vi "I2C Bus Monitor Test.vi"() -> ()   [LabVIEW 2025]
uses:
  b35e104c-1675-4f6f-8f1c-29597b7e93d1.vi
  I2C Bus Monitor UI/I2C Bus Monitor UI.lvlib
  I2C Bus Monitor/I2C Bus Monitor.lvclass
panel:
  out "Count":i32
  in  "Select 2":bool
  in  "SERIAL INPUT (SI)":u32(ring)
  in  "Select":bool
  in  "RESOURCE NAME":u32(ring)
  in  "I2C Scrpit Path":path
  in  "Serial Channel":string(combo)
  in  "Send I2C Script":bool
  out "I2C Script Error":errorcluster
  out "I2C Transaction Error":errorcluster
  in  "I2C Command":T1 {"Data" format="%02x"; "Register Address" format="%04x"; "Slave Address" format="%02x"}
  out "Read Data":u8 format="%02x"
  in  "Send I2C Transaction":bool
  out "User Timestamp Fifo Overflow":bool
  out "i":i32
  out "I2C Messages":string[][](table)
  out "Total Messages":i32
  out "FIFO Pressure":u32
  in  "stop":bool
  out "Bitfile Path":path
  out "SI Count":i32
  out "Module Name":string
  out "error out":errorcluster
  # "takes few seconds to populate"
  # "1"
  # "2"
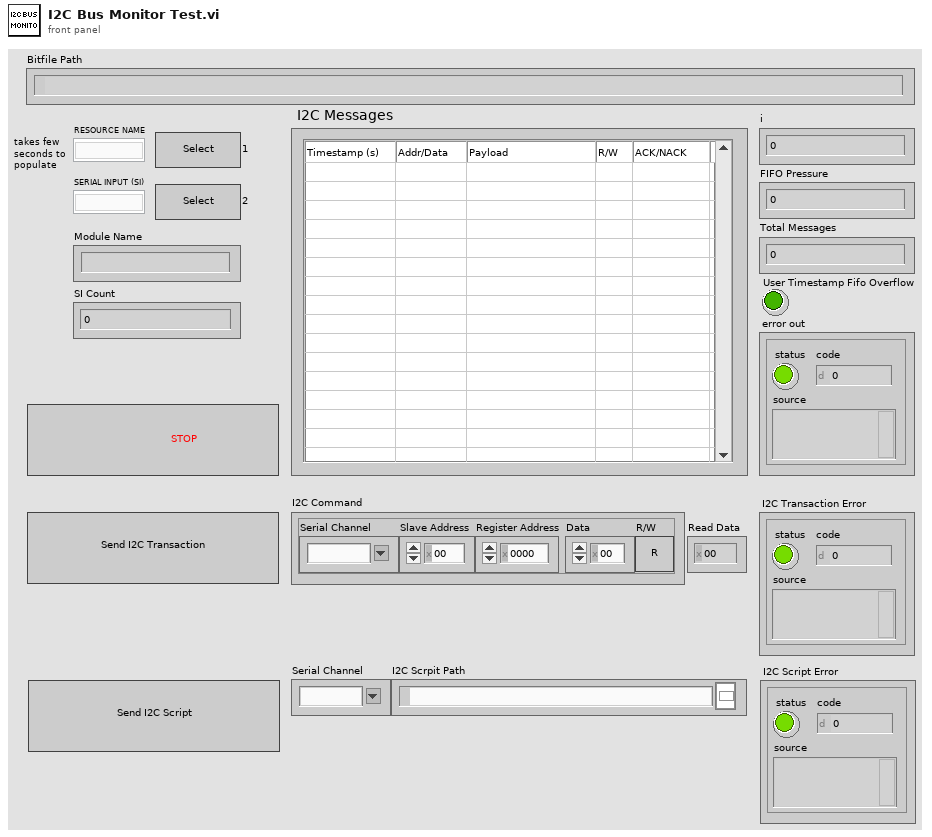
[diagram p1: front panel]
types:
  T1 = cluster{"Serial Channel":string, "Slave Address":u8, "Register Address":u16, "Data":u8, "R/W":bool}
  T2 = typedef "NI CSI-2 API FPGA v2.lvlib/Timestamp ID.ctl" = enum8{"SI0 LLP", "SI1 LLP", "SI2 LLP", "SI3 LLP", "SI4 LLP", "SI5 LLP", "SI6 LLP", "SI7 LLP", "SO0 LLP", "SO1 LLP", "SO2 LLP", "SO3 LLP", "SO4 LLP", "SO5 LLP", "SO6 LLP", "SO7 LLP", "Ser0 GPIO Bank", "Ser1 GPIO Bank", "Ser2 GPIO Bank", "Ser3 GPIO Bank", "Ser4 GPIO Bank", "Ser5 GPIO Bank", "Ser6 GPIO Bank", "Ser7 GPIO Bank", "Des0 GPIO Bank", "Des1 GPIO Bank", "Des2 GPIO Bank", "Des3 GPIO Bank", "Des4 GPIO Bank", "Des5 GPIO Bank", "Des6 GPIO Bank", "Des7 GPIO Bank", "User0", "User1", "User2", "User3", "User4", "User5", "User6", "User7", "User8", "User9", "User10", "User11", "User12", "User13", "User14", "User15", "User16", "User17", "User18", "User19", "User20", "User21", "User22", "User23", "User24", "User25", "User26", "User27", "User28", "User29", "User30", "User31"}
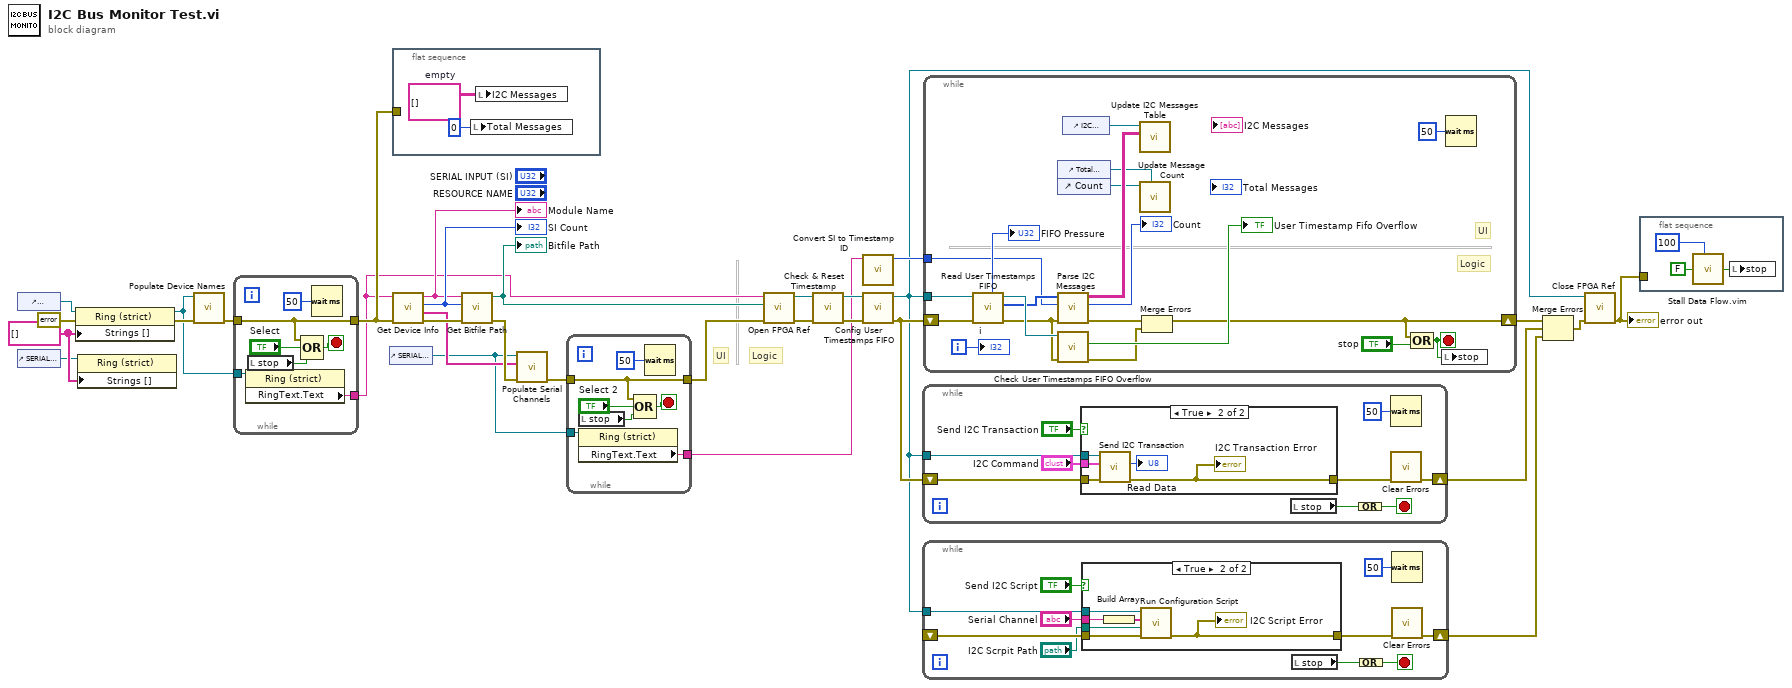
[diagram p0: block diagram]
diagram:
  w2 = string[] [] ("Strings []")
  # "Logic"
  # "UI"
  n1 = control-ref of="RESOURCE NAME"() -> (w4:refnum<vi>)
  n2 = control-ref of="SERIAL INPUT (SI)"() -> (w1:refnum<vi>)
  n3 = property class="Ring (strict)"(reference=w4, error in=errorcluster {"status"=FALSE, "code"=0, "source"=""} ("error constant"), "Strings []"=w2) -> (reference out=w3:refnum<vi>, error out=w5:errorcluster)
  n4 = property class="Ring (strict)"(reference=w1, "Strings []"=w2) -> ()  [unwired: 1 in, 2 out]
  n5 = call "Populate Device Names.vi"("error in (no error)"=w5, "RESOURCE NAME Ref"=w3) -> ("error out"=w14:errorcluster)  [unwired: 8 in, 1 out]
  n6 = while {
    tunnel: [w35] -> w15
    tunnel: w14 -> [w35]
    tunnel: w3 -> [w34]
    tunnel: [w33] -> w6
    stop <- w36 stop-if-true
    n7 = property class="Ring (strict)"(reference=w34) -> ("RingText.Text"=w33:string)  [unwired: 1 in, 2 out]
    n8 = local read "stop"() -> (w32:bool)
    n9 = Compound Arithmetic op=OR(w35, "Select", w32) -> (w36:bool)
    n10 = Wait (ms)(milliseconds to wait=u32 50) -> ()  [unwired: 1 out]
  }
  n11 = control-ref of="SERIAL INPUT (SI)"() -> (w9:refnum<vi>)
  n12 = flat-sequence {
    tunnel: w15 -> [_]
    frame #0 {
      w40 = string[][] []  # empty
      n13 = local write "Total Messages"(0 ("Total Records out")) -> ()
      n14 = local write "I2C Messages"(w40) -> ()
    }
  }
  n15 = call "Get Device Info.vi"("error in (no error)"=w15, "RIO Device"=w6) -> ("error out"=w31:errorcluster, "SI Channels"=w12:string[], "SI Count"=w30:i32, "Module Name"=w13:string)  [unwired: 6 in]
  "Module Name" <- w13
  "SI Count" <- w30
  n16 = call "Get Bitfile Path.vi"("error in (no error)"=w31, "SI Count"=w30, "Module Name"=w13) -> ("error out"=w26:errorcluster, "Bitfile Path"=w29:path)  [unwired: 7 in]
  "Bitfile Path" <- w29
  n17 = call "Populate Serial Channels.vi"("error in (no error)"=w26, "Strings []"=w12, "SERIAL INPUT (SI) Ref in"=w9) -> ("error out"=w11:errorcluster)  [unwired: 7 in, 1 out]
  n18 = while {
    tunnel: [w45] -> w10
    tunnel: w11 -> [w45]
    tunnel: w9 -> [w44]
    tunnel: [w43] -> w7
    stop <- w46 stop-if-true
    n19 = local read "stop"() -> (w41:bool)
    n20 = property class="Ring (strict)"(reference=w44) -> ("RingText.Text"=w43:string)  [unwired: 1 in, 2 out]
    n21 = Compound Arithmetic op=OR(w45, "Select 2", w41) -> (w46:bool)
    n22 = Wait (ms)(milliseconds to wait=u32 50) -> ()  [unwired: 1 out]
  }
  n23 = call "Open FPGA Ref.vi"("error in (no error)"=w10, "Bitfile Path"=w29, "Device address"=w6) -> ("error out"=w28:errorcluster, "FPGA Ref out"=w20:refnum<k20>)  [unwired: 7 in]
  n24 = call "Check & Reset Timestamp.vi"("error in (no error)"=w28, "FPGA Ref in"=w20) -> ("error out"=w21:errorcluster, "FPGA Ref out"=w19:refnum<k20>)  [unwired: 8 in]
  n25 = call "Convert SI to Timestamp ID.vi"("SI Channel"=w7) -> ("Timestamp ID"=w25:T2)  [unwired: 10 in]
  n26 = call "Config User Timestamps FIFO.vi"("error in (no error)"=w21, "FPGA Ref in"=w19) -> ("error out"=w24:errorcluster, "FPGA Ref out"=w18:refnum<k20>)  [unwired: 8 in]
  n27 = while {
    tunnel: w18 -> [w50]
    shift-right: [w48] -> w22
    shift-left: w24 -> [w54]
    stop <- w56 stop-if-true
    n28 = case shown="True" "Send I2C Transaction" {
      tunnel: w54 -> [w57 w62]
      tunnel: [w57 w58] -> w49
      tunnel: "I2C Command" -> [_ w61]
      tunnel: w50 -> [_ w59]
      frame False {
      }
      frame True {
        n29 = call "Send I2C Transaction.vi"("Error In"=w62, "I2C Command"=w61, "FPGA Ref in"=w59) -> ("Error Out"=w58:errorcluster, "Read Data"=→"Read Data":u8)  [unwired: 6 in, 1 out]
        "I2C Transaction Error" <- w58
      }
    }
    n30 = local read "stop"() -> (w55:bool)
    n31 = Compound Arithmetic op=OR(w55) -> (w56:bool)
    n32 = Wait (ms)(milliseconds to wait=u32 50) -> ()  [unwired: 1 out]
    n33 = call <vilib>:"Clear Errors.vi"("error in (no error)"=w49) -> ("error out"=w48:errorcluster)  [unwired: 5 in, 1 out]
  }
  n34 = while {
    shift-right: [w66] -> w17
    shift-left: _ -> [w70]
    tunnel: w18 -> [w65]
    stop <- w72 stop-if-true
    n35 = case shown="True" "Send I2C Script" {
      tunnel: w70 -> [w73 w79]
      tunnel: [w73 w77] -> w67
      tunnel: w65 -> [_ w78]
      tunnel: "I2C Scrpit Path" -> [_ w76]
      tunnel: "Serial Channel" -> [_ w75]
      frame False {
      }
      frame True {
        n36 = Build Array(w75) -> (w74:string[])
        n37 = call "Run Configuration Script.vi"("error in (no error)"=w79, "configuration script"=w76, "serial channels"=w74, "fpga interface in"=w78) -> ("error out"=w77:errorcluster)  [unwired: 6 in, 1 out]
        "I2C Script Error" <- w77
      }
    }
    n38 = local read "stop"() -> (w71:bool)
    n39 = Compound Arithmetic op=OR(w71) -> (w72:bool)
    n40 = Wait (ms)(milliseconds to wait=u32 50) -> ()  [unwired: 1 out]
    n41 = call <vilib>:"Clear Errors.vi"("error in (no error)"=w67) -> ("error out"=w66:errorcluster)  [unwired: 5 in, 1 out]
  }
  n42 = while {
    shift-right: [w86] -> w27
    shift-left: w24 -> [w97]
    tunnel: w25 -> [w83]
    tunnel: w18 -> [w98]
    i -> [w96]
    stop <- w84 stop-if-true
    # "Logic"
    # "UI"
    n43 = call "Read User Timestamps FIFO.vi"("error in (no error)"=w97, "FPGA Ref in"=w98) -> ("error out"=w89:errorcluster, "Data"=w90:u64[], "FPGA Ref out"=w93:refnum<k20>, "Elements Remaining"=→"FIFO Pressure":u32)  [unwired: 6 in]
    n44 = control-ref of="Total Messages"() -> (w82:refnum<vi>)
    n45 = control-ref of="Count"() -> (w80:refnum<vi>)
    n46 = call "Parse I2C Messages.vi"("error in (no error)"=w89, "Timestamp ID"=w83, "User Timestamps"=w90) -> ("error out"=w88:errorcluster, "Count"=→"Count":i32, "I2C Messages"=w85:string[][])  [unwired: 6 in]
    n47 = call "Check User Timestamps FIFO Overflow.vi"("error in (no error)"=w89, "FPGA Ref in"=w93) -> ("error out"=w87:errorcluster, "User Timestamp FIFO Overflow"=→"User Timestamp Fifo Overflow":bool)  [unwired: 7 in, 1 out]
    n48 = control-ref of="I2C Messages"() -> (w91:refnum<vi>)
    n49 = call "Update I2C Messages Table.vi"("I2C Messages in"=w85, "I2C Table Ref"=w91) -> ()  [unwired: 9 in, 1 out]
    n50 = call "Update Message Count.vi"("I2C Messages Count Ref"=w82, "Fetch Count Ref"=w80) -> ()  [unwired: 9 in, 1 out]
    n51 = Merge Errors(w88, w87) -> (w86:errorcluster)
    n52 = Compound Arithmetic op=OR(w86, "stop") -> (w84:bool)
    n53 = local write "stop"(w84) -> ()
    n54 = Wait (ms)(milliseconds to wait=u32 50) -> ()  [unwired: 1 out]
    "i" <- w96
  }
  n55 = Merge Errors(w27, w22, w17) -> (w23:errorcluster)
  n56 = call "Close FPGA Ref.vi"("error in (no error)"=w23, "FPGA Ref in"=w18) -> ("error out"=w8:errorcluster)  [unwired: 9 in]
  "error out" <- w8
  n57 = flat-sequence {
    tunnel: w8 -> [_]
    frame #0 {
      n58 = call "Stall Data Flow.vim"("value in"=FALSE ("stop"), "milliseconds to wait"=u32 100) -> ("value out"=w101:bool)  [unwired: 1 out]
      n59 = local write "stop"(w101) -> ()
    }
  }
